vi "Seq Test Editor.vi"(6 "User Name":string="Jon", 8 "Sys Error":errorcluster, 9 "Part Type":string="LX", 10 "Station":string="Audit Station", 11 "Base Path":path=path "C:/Labview Code") -> (0 "Sys Error Out":errorcluster)   [LabVIEW 2018]
uses:
  type defs/Sequence Info.ctl
  type defs/Sequence Status.ctl
  type defs/config paths for seq def.ctl
  <vilib>/Utility/miscctls.llb/LVRowAndColumnUnsignedTypeDef.ctl
  <vilib>/Utility/file.llb/Write To Spreadsheet File (string).vi
panel:
  in  "Save":bool
  out "Sequence Name":string="F15 Audit 1 Sequence"
  in  "Exit":bool
  in  "Sequence":i32(listbox)=7
  in  "Steps":i32(listbox)
  in  "Edit Step":bool
  in  "Up":bool
  in  "Down":bool
  in  "Copy Step":bool
  in  "Delete":bool
  in  "Insert Step":bool
  # "[Page Up]"
  # "[Page Dn]"
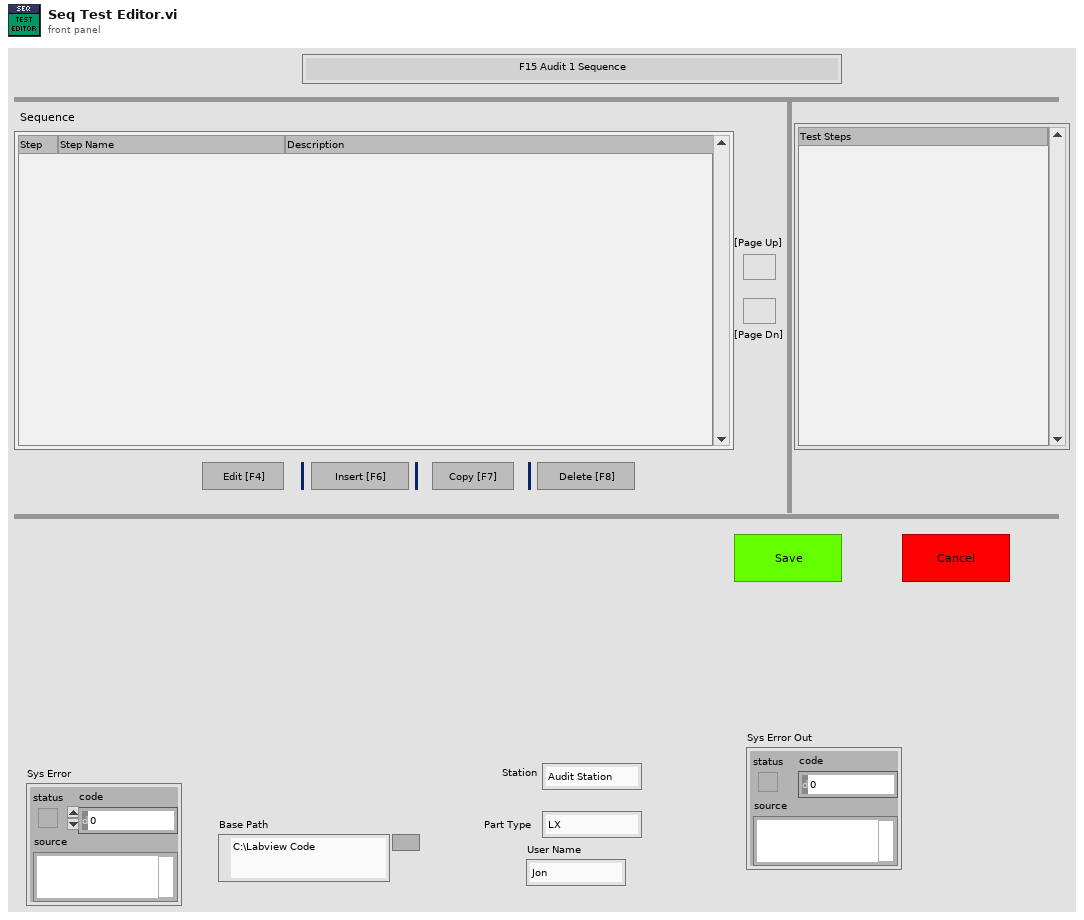
[diagram p1: front panel]
types:
  T1 = typedef "Sequence Status.ctl" = enum16{"No Change", "Edited", "New Step", "Deleted", "Moved Up", "Moved Down", "Copied"}
  T2 = typedef "Sequence Info.ctl" = cluster{"Name":string, "Description":string, "data string":string}
  T3 = cluster{"Type":string, "Sequence Name:":i32, "Sequence":refnum<vi>, "Steps":refnum<vi>, "Sequence Info":T2[], "Sequence Scroll":u32, "Basic Steps":string[], "Sequences":string[], "Sequence Text":string, "appended path":path, "Station":string, "New Step?":bool, "Part Type":string, "User Name":string, "Sequence History":string[][], "Sequence Status":T1, "Sequence History Index":i32, "Step History Data":string[], "VI Names":string[], "Sys Error":errorcluster, "Current Sequence":string[][], "Sequence Path":path, "Base Path":path}
  T4 = enum8{"Enabled", "Disabled", "Disabled and Grayed Out"}
  T5 = typedef "config paths for seq def.ctl" = cluster{"Part Type":string, "base path":path}
  T6 = typedef "LVRowAndColumnUnsignedTypeDef.ctl" = cluster{"Row":u32, "Column":u32}
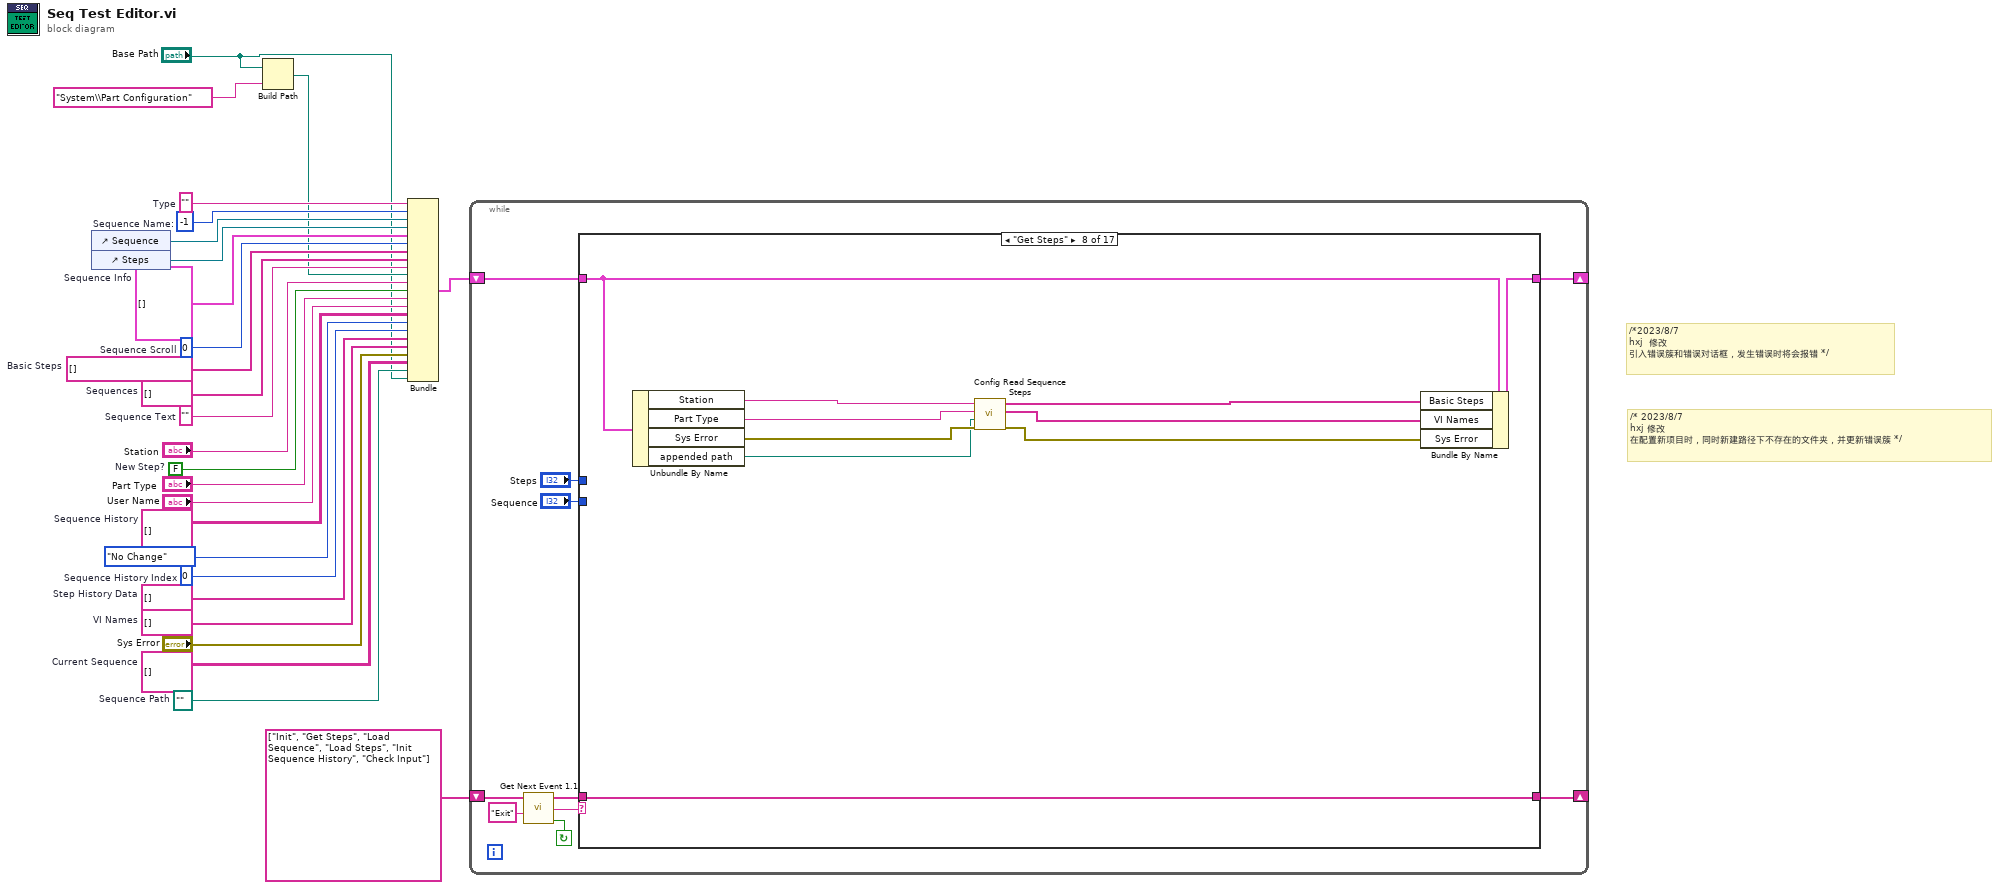
[diagram p0: block diagram]
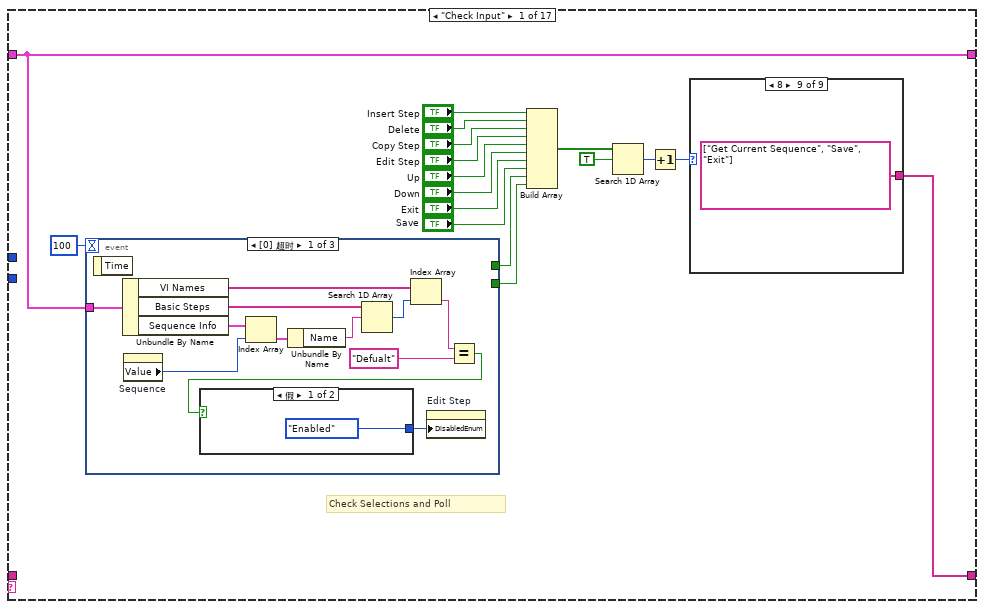
[diagram p2: hidden frame]
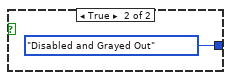
[diagram p3: hidden frame]
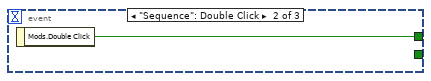
[diagram p4: hidden frame]
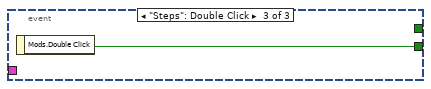
[diagram p5: hidden frame]
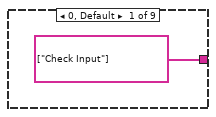
[diagram p6: hidden frame]
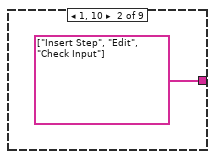
[diagram p7: hidden frame]
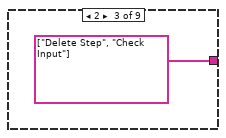
[diagram p8: hidden frame]
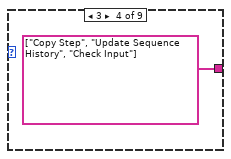
[diagram p9: hidden frame]
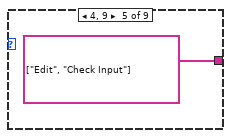
[diagram p10: hidden frame]
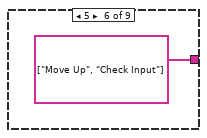
[diagram p11: hidden frame]
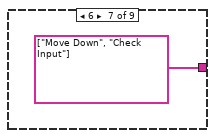
[diagram p12: hidden frame]
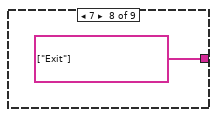
[diagram p13: hidden frame]
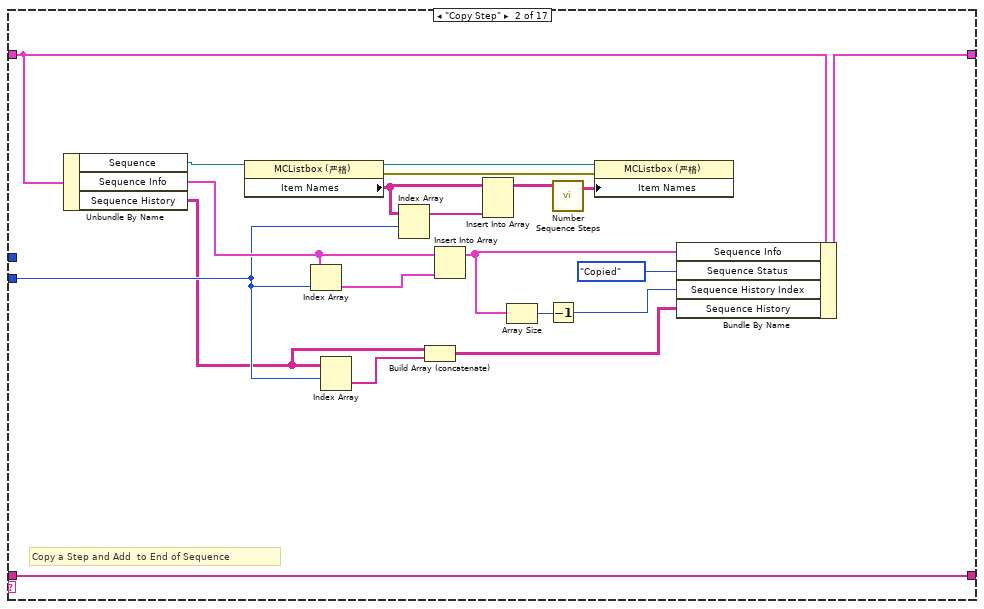
[diagram p14: hidden frame]
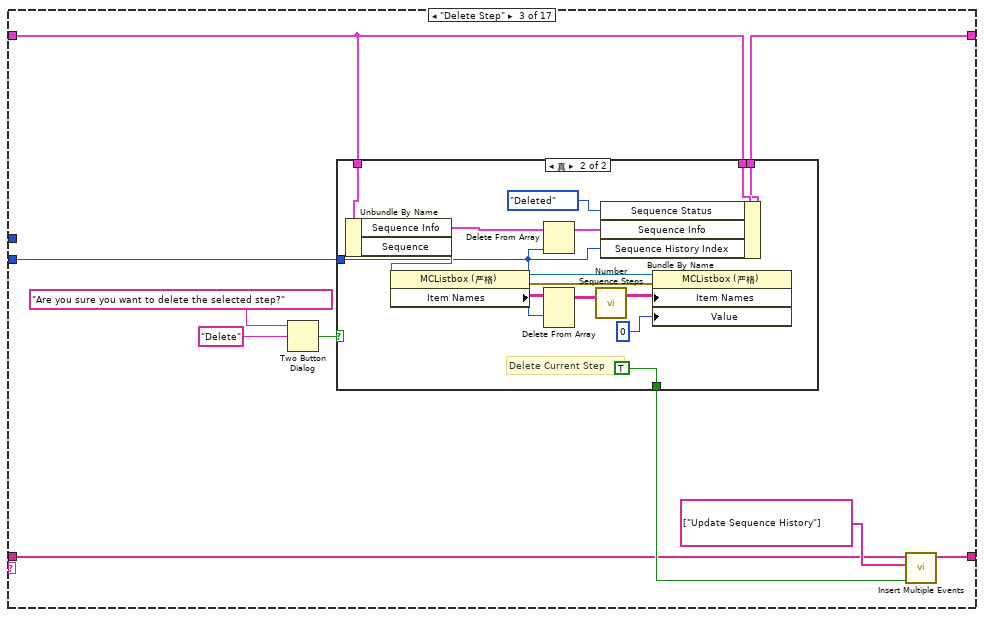
[diagram p15: hidden frame]
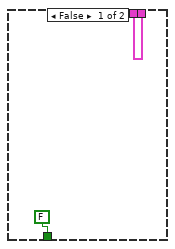
[diagram p16: hidden frame]
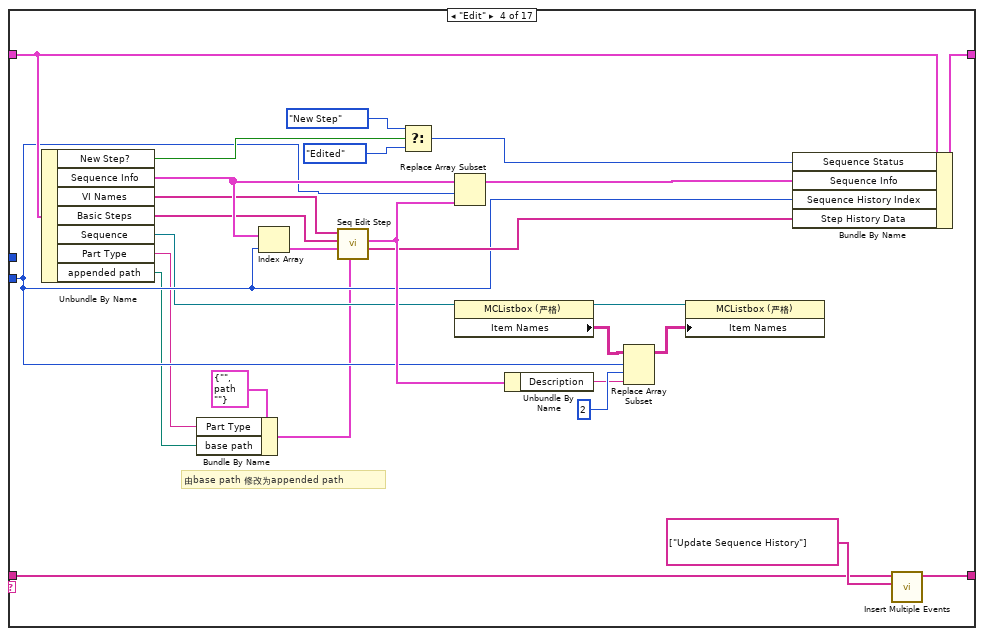
[diagram p17: hidden frame]
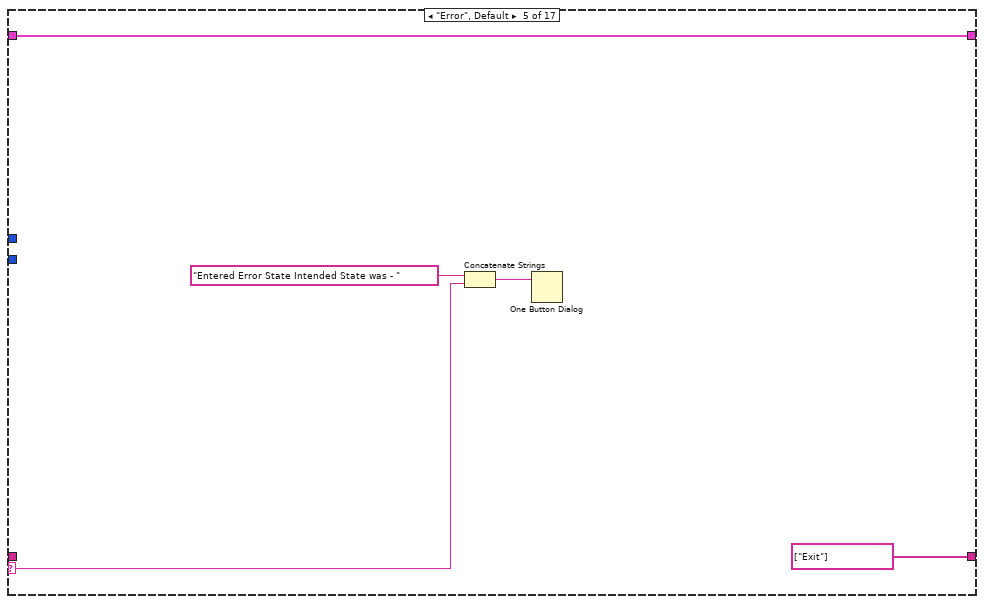
[diagram p18: hidden frame]
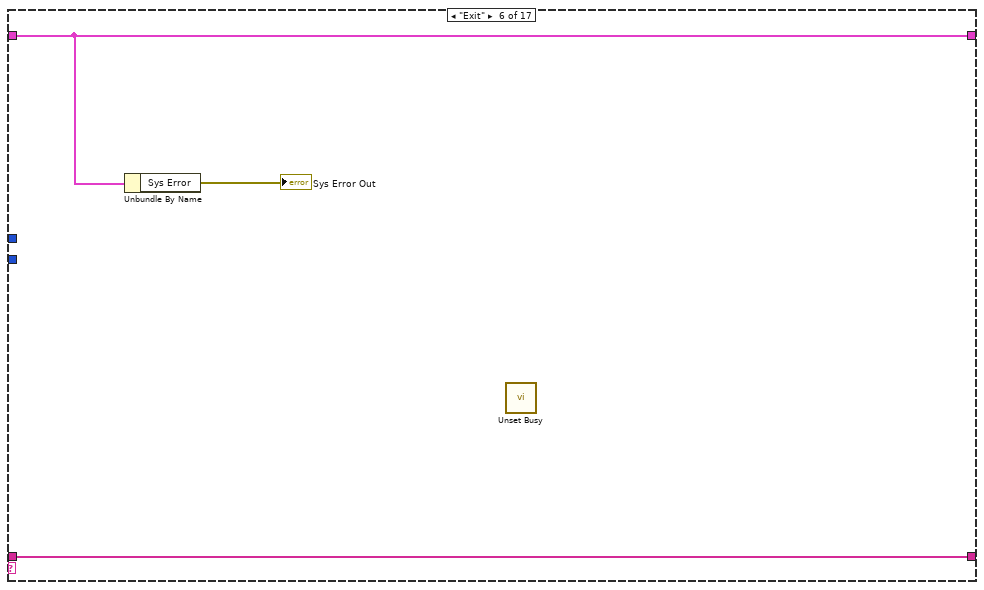
[diagram p19: hidden frame]
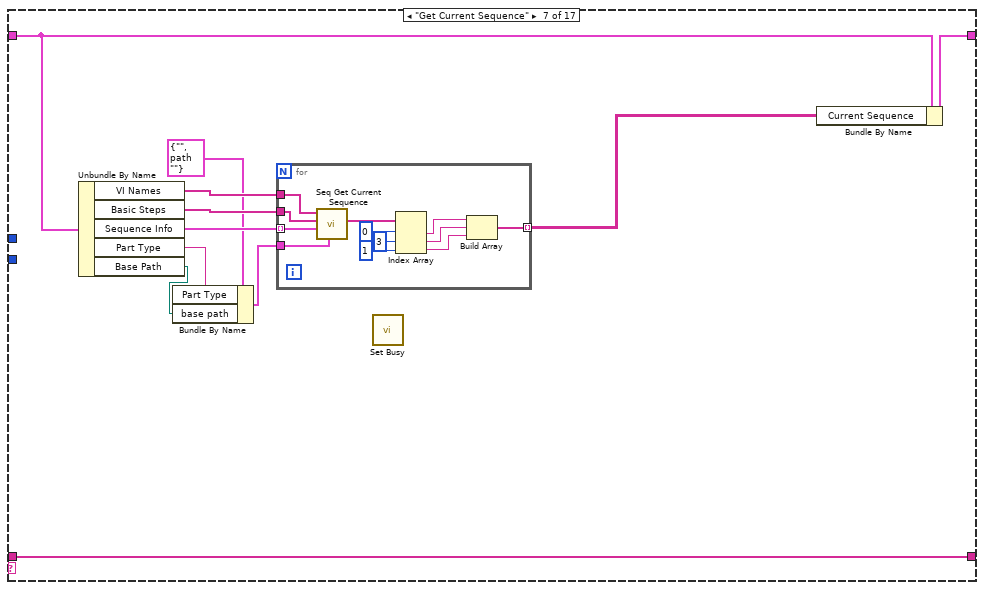
[diagram p20: hidden frame]
diagram:
  w4 = path ""  # Sequence Path
  w5 = string[][] []  # Current Sequence
  w7 = string[] []  # VI Names
  w8 = string[] []  # Step History Data
  w9 = 0  # Sequence History Index
  w16 = FALSE  # New Step?
  w11 = string[][] []  # Sequence History
  w14 = T2[] []  # Sequence Info
  w18 = string[] []  # Sequences
  w20 = ""  # Sequence Text
  w21 = -1  # Sequence Name:
  w17 = string[] []  # Basic Steps
  w23 = u32 0  # Sequence Scroll
  w19 = ""  # Type
  # "/* 2023/8/7\nhxj 修改\n在配置新项目时，同时新建路径下不存在的文件夹，并更新错误簇 */"
  # "/*2023/8/7\nhxj  修改\n引入错误簇和错误对话框，发生错误时将会报错 */"
  n1 = control-ref of="Sequence"() -> (w24:refnum<vi>)
  n2 = control-ref of="Steps"() -> (w22:refnum<vi>)
  n3 = Build Path(base path="Base Path", name or relative path="System\\Part Configuration" ("string")) -> (appended path=w3:path)
  n4 = Bundle("Type"=w19, "Sequence Name:"=w21, "Sequence"=w24, "Steps"=w22, "Sequence Info"=w14, "Sequence Scroll"=w23, "Basic Steps"=w17, "Sequences"=w18, "Sequence Text"=w20, "appended path"=w3, "Station"="Station", "New Step?"=w16, "Part Type"="Part Type", "User Name"="User Name", "Sequence History"=w11, "Sequence Status"=Sequence_Status."No Change", "Sequence History Index"=w9, "Step History Data"=w8, "VI Names"=w7, "Sys Error"="Sys Error", "Current Sequence"=w5, "Sequence Path"=w4, "Base Path"="Base Path") -> (w25:T3)  [unwired: 1 in]
  n5 = while {
    shift-right: [w36] -> _
    shift-left: string[] ["Init", "Get Steps", "Load Sequence", "Load Steps", "Init Sequence History", "Check Input"] -> [w33]
    shift-right: [w34] -> _
    shift-left: w25 -> [w35]
    stop <- w30 continue-if-true
    n6 = call "Get Next Event 1.1.vi"("Exit Event"="Exit", "event queue in"=w33) -> ("Condition (Exit:F)"=w30:bool, "next event"=w31:string, "event queue out"=w32:string[])  [unwired: 6 in, 1 out]
    n7 = case shown="\"Get Steps\"" w31 {
      selector: w31 -> [_ _ _ _ w154 _ _ _ _ _ _ _ _ _ _ _ _]
      tunnel: w32 -> [_ w91 w99 w133 _ w160 w171 w193 w202 w217 w230 w265 w273 w275 w311 w346 w402]
      tunnel: [w46 w91 w100 w134 string[] ["Exit"] ("event queue out") w160 w171 w193 w202 w217 w230 w265 w273 w276 w310 w346 w402] -> w36
      tunnel: w35 -> [w37 w93 w105 w152 w157 w159 w167 w192 w196 w207 w241 w263 w268 w286 w313 w338 w399]
      tunnel: [w37 w92 w104 w151 w157 w159 w166 w191 w196 w206 w240 w267 w268 w288 w315 w337 w401] -> w34
      tunnel: "Steps" -> [_ _ _ _ _ _ _ _ _ _ w234 _ _ _ _ _ _]
      tunnel: "Sequence" -> [_ w83 w103 w136 _ _ _ _ _ _ w229 _ _ w280 w314 _ _]
      frame "Check Input" {
        # "Check Selections and Poll"
        n8 = event shown="[0] 超时" {
          selector: _ -> [_ _ _]
          dyn-events: _ -> [_ _ _]
          timeout: 100 -> [_ _ _]
          tunnel: [_ w68 _] -> w43
          tunnel: [_ _ w69] -> w42
          tunnel: w37 -> [w65 _ _]
          event Timeout {
            n9 = event-data() -> ()  [unwired: 1 in, 1 out]
            n10 = Unbundle By Name(w65) -> ("VI Names"=w60:string[], "Basic Steps"=w62:string[], "Sequence Info"=w64:T2[])
            n11 = property on="Sequence" class="MCListbox (严格)"() -> ("Value"=w54:i32)  [unwired: 2 in, 2 out]
            n12 = Index Array(array=w64, index=w54) -> (element=w63:T2)
            n13 = Unbundle By Name(w63) -> ("Name"=w61:string)
            n14 = Search 1D Array(1D array=w62, element=w61) -> (index of element=w59:i32)  [unwired: 1 in]
            n15 = Index Array(array=w60, index=w59) -> (element=w57:string)
            n16 = Equal?(x=w57, y="Defualt") -> (x = y?=w56:bool)
            n17 = case shown="假" w56 {
              tunnel: [T4."Enabled" ("禁用") T4."Disabled and Grayed Out" ("禁用")] -> w55
              frame False {
              }
              frame True {
              }
            }
            n18 = property on="Edit Step" class="Bool"("DisabledEnum"=w55) -> ()  [unwired: 2 in, 2 out]
          }
          event "Sequence": Double Click {
            n19 = event-data() -> ("Mods.Double Click"=w68:bool)  [unwired: 1 in]
          }
          event "Steps": Double Click {
            n20 = event-data() -> ("Mods.Double Click"=w69:bool)  [unwired: 1 in]
          }
        }
        n21 = Build Array("Insert Step", "Delete", "Copy Step", "Edit Step", "Up", "Down", "Exit", "Save", w43, w42) -> (w49:bool[])
        n22 = Search 1D Array(1D array=w49, element=TRUE) -> (index of element=w48:i32)  [unwired: 1 in]
        n23 = Increment(x=w48) -> (x+1=w38:i32)
        n24 = case shown="8" w38 {
          tunnel: [string[] ["Check Input"] string[] ["Insert Step", "Edit", "Check Input"] string[] ["Delete Step", "Check Input"] string[] ["Copy Step", "Update Sequence History", "Check Input"] string[] ["Edit", "Check Input"] string[] ["Move Up", "Check Input"] string[] ["Move Down", "Check Input"] string[] ["Exit"] string[] ["Get Current Sequence", "Save", "Exit"]] -> w46
          frame 0, Default {
          }
          frame 1, 10 {
          }
          frame 2 {
          }
          frame 3 {
          }
          frame 4, 9 {
          }
          frame 5 {
          }
          frame 6 {
          }
          frame 7 {
          }
          frame 8 {
          }
        }
      }
      frame "Copy Step" {
        # "Copy a Step and Add  to End of Sequence"
        n25 = Unbundle By Name(w93) -> ("Sequence"=w98:refnum<vi>, "Sequence Info"=w88:T2[], "Sequence History"=w82:string[][])
        n26 = property class="MCListbox (严格)"(reference=w98) -> (reference out=w95:refnum<vi>, error out=w94:errorcluster, "Item Names"=w90:string[][])  [unwired: 1 in]
        n27 = Index Array(array=w88, index=w83) -> (element=w87:T2)
        n28 = Index Array(array=w82, index (row)=w83) -> (element=w81:string[])  [unwired: 1 in]
        n29 = Index Array(array=w90, index (row)=w83) -> (element=w89:string[])  [unwired: 1 in]
        n30 = Build Array (concatenate)(w82, w81) -> (w80:string[][])
        n31 = Insert Into Array(array=w88, new element=w87) -> (w79:T2[])  [unwired: 1 in]
        n32 = Insert Into Array(array=w90, new element=w89) -> (w97:string[][])  [unwired: 2 in]
        n33 = Array Size(array=w79) -> (size(s)=w85:i32)
        n34 = Decrement(x=w85) -> (x-1=w84:i32)
        n35 = call "Number Sequence Steps.vi"("Sequence Names"=w97) -> ("ItemNames Out"=w96:string[][])  [unwired: 1 out]
        n36 = property class="MCListbox (严格)"(reference=w95, error in=w94, "Item Names"=w96) -> ()  [unwired: 2 out]
        n37 = Bundle By Name(cluster=w93, "Sequence Info"=w79, "Sequence Status"=Sequence_Status."Copied", "Sequence History Index"=w84, "Sequence History"=w80) -> (w92:T3)
      }
      frame "Delete Step" {
        n38 = Two Button Dialog(message="Are you sure you want to delete the selected step?", 2:"Delete" ("T button name (\"OK\")")) -> (T button?=w106:bool)  [unwired: 1 in]
        n39 = case shown="真" w106 {
          tunnel: w105 -> [_ w125]
          tunnel: w105 -> [w110 w123]
          tunnel: [w110 w122] -> w104
          tunnel: w103 -> [_ w112]
          tunnel: [FALSE TRUE] -> w101
          frame False {
          }
          frame True {
            # "Delete Current Step"
            n40 = Unbundle By Name(w125) -> ("Sequence Info"=w121:T2[], "Sequence"=w124:refnum<vi>)
            n41 = property class="MCListbox (严格)"(reference=w124) -> (reference out=w118:refnum<vi>, error out=w117:errorcluster, "Item Names"=w119:string[][])  [unwired: 1 in]
            n42 = Delete From Array(array=w121, index=w112) -> (array with subset deleted=w120:T2[])  [unwired: 1 in, 1 out]
            n43 = Delete From Array(array=w119, index (row)=w112) -> (array with subset deleted=w116:string[][])  [unwired: 2 in, 1 out]
            n44 = call "Number Sequence Steps.vi"("Sequence Names"=w116) -> ("ItemNames Out"=w115:string[][])  [unwired: 1 out]
            n45 = Bundle By Name(cluster=w123, "Sequence Status"=Sequence_Status."Deleted", "Sequence Info"=w120, "Sequence History Index"=w112) -> (w122:T3)
            n46 = property class="MCListbox (严格)"(reference=w118, error in=w117, "Item Names"=w115, "Value"=0) -> ()  [unwired: 2 out]
          }
        }
        n47 = call "Insert Multiple Events.vi"("Insert all? (T)"=w101, "Events to Insert"=string[] ["Update Sequence History"], "Event queue in"=w99) -> ("Event queue out"=w100:string[])  [unwired: 4 in]
      }
      frame "Edit" {
        # "由base path 修改为appended path"
        n48 = Unbundle By Name(w152) -> ("New Step?"=w141:bool, "Sequence Info"=w149:T2[], "VI Names"=w132:string[], "Basic Steps"=w130:string[], "Sequence"=w131:refnum<vi>, "Part Type"=w128:string, "appended path"=w126:path)
        n49 = Bundle By Name(cluster=T5 {"Part Type"="", "base path"=path ""} ("config paths"), "Part Type"=w128, "base path"=w126) -> (w127:T5)
        n50 = Index Array(array=w149, index=w136) -> (element=w142:T2)
        n51 = call "Seq Edit Step.vi"("config paths"=w127, "Segment Info In"=w142, "Basic Steps"=w130, "VI Names"=w132) -> ("Step Hisitory"=w137:string[], "Segment Info Out"=w148:T2)  [unwired: 4 in, 2 out]
        n52 = Select(t=Sequence_Status."New Step" ("Sequence Status"), s=w141, f=Sequence_Status."Edited" ("Sequence Status")) -> (s? t:f=w138:T1)
        n53 = Replace Array Subset(array=w149, new element=w148, index=w136) -> (w150:T2[])
        n54 = property class="MCListbox (严格)"(reference=w131) -> (reference out=w146:refnum<vi>, "Item Names"=w147:string[][])  [unwired: 1 in, 1 out]
        n55 = Unbundle By Name(w148) -> ("Description"=w144:string)
        n56 = Replace Array Subset(array=w147, new element=w144, index (row)=w136, index (col)=2 ("disabled index (col)")) -> (w143:string[][])
        n57 = property class="MCListbox (严格)"(reference=w146, "Item Names"=w143) -> ()  [unwired: 1 in, 2 out]
        n58 = Bundle By Name(cluster=w152, "Sequence Status"=w138, "Sequence Info"=w150, "Sequence History Index"=w136, "Step History Data"=w137) -> (w151:T3)
        n59 = call "Insert Multiple Events.vi"("Events to Insert"=string[] ["Update Sequence History"], "Event queue in"=w133) -> ("Event queue out"=w134:string[])  [unwired: 5 in]
      }
      frame "Error", Default {
        n60 = Concatenate Strings("Entered Error State Intended State was - " ("string"), w154) -> (w153:string)
        n61 = One Button Dialog(message=w153) -> ()  [unwired: 1 in, 1 out]
      }
      frame "Exit" {
        n62 = Unbundle By Name(w159) -> ("Sys Error"=→"Sys Error Out":errorcluster)
        n63 = call <vilib>:"Unset Busy.vi"() -> ()  [unwired: 11 in, 1 out]
      }
      frame "Get Current Sequence" {
        n64 = Unbundle By Name(w167) -> ("VI Names"=w168:string[], "Basic Steps"=w169:string[], "Sequence Info"=w170:T2[], "Part Type"=w163:string, "Base Path"=w162:path)
        n65 = Bundle By Name(cluster=T5 {"Part Type"="", "base path"=path ""} ("config paths"), "Part Type"=w163, "base path"=w162) -> (w161:T5)
        n66 = for {
          tunnel: w170 -> [w183] mode=indexing
          tunnel: w169 -> [w182]
          tunnel: w168 -> [w181]
          tunnel: [w176] -> w165 mode=indexing
          tunnel: w161 -> [w172]
          n67 = call "Seq Get Current Sequence.vi"("config paths"=w172, "Segment Info In"=w183, "Basic Steps"=w182, "VI Names"=w181) -> ("Step Hisitory"=w180:string[])  [unwired: 6 in, 1 out]
          n68 = Index Array(array=w180, index #1=0 ("index"), index #2=3 ("index"), index #3=1 ("index")) -> (element #1=w179:string, element #2=w178:string, element #3=w177:string)
          n69 = Build Array(w179, w178, w177) -> (w176:string[])
        }
        n70 = call <vilib>:"Set Busy.vi"() -> ()  [unwired: 10 in, 2 out]
        n71 = Bundle By Name(cluster=w167, "Current Sequence"=w165) -> (w166:T3)
      }
      frame "Get Steps" {
        n72 = Unbundle By Name(w192) -> ("Station"=w189:string, "Part Type"=w190:string, "Sys Error"=w186:errorcluster, "appended path"=w184:path)
        n73 = call "Config Read Sequence Steps.vi"("Error In"=w186, "Base Path"=w184, "Part Type"=w190, "Station Name"=w189) -> ("Error Out"=w185:errorcluster, "VI Names"=w187:string[], "Sequence Steps"=w188:string[])  [unwired: 5 in]
        n74 = Bundle By Name(cluster=w192, "Basic Steps"=w188, "VI Names"=w187, "Sys Error"=w185) -> (w191:T3)
      }
      frame "Init" {
        w199 = string[][] [] ("Item Names")
        w198 = u32 0
        w195 = 0 ("Value")
        n75 = Unbundle By Name(w196) -> ("Sequence"=w201:refnum<vi>, "Steps"=w200:refnum<vi>)
        n76 = property class="MCListbox (严格)"(reference=w201, "Item Names"=w199, "Value"=w195, "Selection Color"=w198) -> ()  [unwired: 1 in, 2 out]
        n77 = property class="MCListbox (严格)"(reference=w200, "Item Names"=w199, "Value"=w195, "Selection Color"=w198, "Disabled Items"=i32[] [], "TopLeft"=T6 {"Row"=0, "Column"=0} ("左上可见单元格")) -> ()  [unwired: 1 in, 2 out]
      }
      frame "Init Sequence History" {
        n78 = Unbundle By Name(w207) -> ("User Name"=w211:string, "Part Type"=w213:string, "Station"=w215:string, "Sequence Info"=w216:T2[], "Sequence Status"=w204:T1)
        n79 = Get Date/Time String() -> (date string=w209:string, time string=w210:string)  [unwired: 3 in]
        n80 = Format Into String(w213) -> (resulting string=w212:string)  [unwired: 3 in, 1 out]
        n81 = Format Into String(w215) -> (resulting string=w214:string)  [unwired: 3 in, 1 out]
        n82 = Format Into String(w204) -> (resulting string=w208:string)  [unwired: 3 in, 1 out]
        n83 = for {
          tunnel: w216 -> [w227] mode=indexing
          tunnel: w214 -> [w222]
          tunnel: w212 -> [w223]
          tunnel: w211 -> [w224]
          tunnel: w210 -> [w225]
          tunnel: w209 -> [w226]
          tunnel: [w220] -> w205 mode=indexing
          tunnel: w208 -> [w219]
          tunnel: "NA" -> [w218]
          n84 = Unbundle By Name(w227) -> ("Name"=w221:string)
          n85 = Build Array(w224, w226, w225, w223, w222, w221, w219, w218, w218) -> (w220:string[])
        }
        n86 = Bundle By Name(cluster=w207, "Sequence History"=w205) -> (w206:T3)
      }
      frame "Insert Step" {
        n87 = Unbundle By Name(w241) -> ("Sequence"=w249:refnum<vi>, "Steps"=w252:refnum<vi>, "Sequence Info"=w236:T2[])
        n88 = property class="MCListbox (严格)"(reference=w252) -> (error out=w248:errorcluster, "Item Names"=w251:string[][])  [unwired: 1 in, 1 out]
        n89 = case shown="..-1" w229 {
          selector: w229 -> [w253 _]
          tunnel: [w253 0 ("Sequence")] -> w228
          frame 0.. {
          }
          frame ..-1 {
          }
        }
        n90 = Index Array(array=w251, index (row)=w234, index (col)=0 ("disabled index (col)")) -> (element=w235:string)
        n91 = property class="MCListbox (严格)"(reference=w249, error in=w248) -> (reference out=w243:refnum<vi>, error out=w242:errorcluster, "Item Names"=w246:string[][])
        n92 = Bundle By Name(cluster=T2 {"Name"="", "Description"="", "data string"=""} ("Segment Data"), "Name"=w235) -> (w238:T2)
        n93 = Build Array("1" ("element"), w235, "") -> (w245:string[])
        n94 = Insert Into Array(array=w246, index (row)=w228, new element=w245) -> (w247:string[][])  [unwired: 1 in]
        n95 = Insert Into Array(array=w236, index=w228, new element=w238) -> (w237:T2[])
        n96 = call "Number Sequence Steps.vi"("Sequence Names"=w247) -> ("ItemNames Out"=w244:string[][])  [unwired: 1 out]
        n97 = property class="MCListbox (严格)"(reference=w243, error in=w242, "Item Names"=w244, "Value"=w228) -> ()  [unwired: 2 out]
        n98 = Bundle By Name(cluster=w241, "Sequence Info"=w237, "New Step?"=TRUE) -> (w240:T3)
      }
      frame "Load Sequence" {
        # "Load Sequence"
        n99 = Unbundle By Name(w263) -> ("Sequence"=w266:refnum<vi>, "Part Type"=w259:string, "Station"=w260:string, "appended path"=w257:path, "Sys Error"=w256:errorcluster)
        n100 = call "Config Load Sequence.vi"("Sys Error In"=w256, "Base Path"=w257, "Station"=w260, "Part Type"=w259) -> ("Sys Error Out"=w255:errorcluster, "Sequence Name"=→"Sequence Name":string, "Item Names"=w264:string[][], "Seqence Info"=w262:T2[], "Sequence Path"=w258:path)  [unwired: 3 in]
        n101 = property class="MCListbox (严格)"(reference=w266, "Item Names"=w264) -> ()  [unwired: 1 in, 2 out]
        n102 = Bundle By Name(cluster=w263, "Sequence Path"=w258, "Sequence Info"=w262, "Sys Error"=w255) -> (w267:T3)
      }
      frame "Load Steps" {
        n103 = Unbundle By Name(w268) -> ("Steps"=w272:refnum<vi>, "Basic Steps"=w271:string[])
        n104 = Build Array(w271) -> (w270:string[][])
        n105 = Transpose 2D Array(2D array=w270) -> (transposed array=w269:string[][])
        n106 = property class="MCListbox (严格)"(reference=w272, "Item Names"=w269) -> ()  [unwired: 1 in, 2 out]
      }
      frame "Move Down" {
        # "Move the step Down one in the sequence"
        n107 = Unbundle By Name(w286) -> ("Sequence Info"=w285:T2[], "Sequence"=w284:refnum<vi>)
        n108 = property class="MCListbox (严格)"(reference=w284) -> (reference out=w289:refnum<vi>, error out=w287:errorcluster, "Item Names"=w283:string[][])  [unwired: 1 in]
        n109 = Array Size(array=w283) -> (size(s)=w282:i32[])
        n110 = Index Array(array=w282) -> (element=w281:i32)  [unwired: 1 in]
        n111 = Decrement(x=w281) -> (x-1=w278:i32)
        n112 = Greater?(x=w278, y=w280) -> (0:w279:bool)
        n113 = case shown="假" w279 {
          tunnel: w289 -> [_ w308]
          tunnel: [w291 w307] -> w288
          tunnel: w287 -> [_ w306]
          tunnel: w286 -> [w291 w305]
          tunnel: w285 -> [_ w304]
          tunnel: w283 -> [_ w300]
          tunnel: w280 -> [_ w293]
          tunnel: [FALSE TRUE] -> w274
          frame False {
            # "At Bottom"
          }
          frame True {
            # "Move Down"
            n114 = Delete From Array(array=w304, index=w293) -> (deleted portion=w302:T2, array with subset deleted=w303:T2[])  [unwired: 1 in]
            n115 = Delete From Array(array=w300, index (row)=w293) -> (deleted portion=w298:string[], array with subset deleted=w299:string[][])  [unwired: 2 in]
            n116 = Increment(x=w293) -> (x+1=w297:i32)
            n117 = Insert Into Array(array=w303, index=w297, new element=w302) -> (w301:T2[])
            n118 = Insert Into Array(array=w299, index (row)=w297, new element=w298) -> (w296:string[][])  [unwired: 1 in]
            n119 = Bundle By Name(cluster=w305, "Sequence Status"=Sequence_Status."Moved Down", "Sequence Info"=w301, "Sequence History Index"=w293) -> (w307:T3)
            n120 = call "Number Sequence Steps.vi"("Sequence Names"=w296) -> ("ItemNames Out"=w295:string[][])  [unwired: 1 out]
            n121 = property class="MCListbox (严格)"(reference=w308, error in=w306, "Item Names"=w295, "Value"=w297) -> ()  [unwired: 2 out]
          }
        }
        n122 = call "Insert Multiple Events.vi"("Insert all? (T)"=w274, "Events to Insert"=string[] ["Update Sequence History"], "Event queue in"=w275) -> ("Event queue out"=w276:string[])  [unwired: 4 in]
      }
      frame "Move Up" {
        # "Move the Step Up one in the Sequence"
        n123 = case shown="1, 默认" w314 {
          selector: w314 -> [_ w319]
          tunnel: [w317 w335] -> w315
          tunnel: w313 -> [w317 w325]
          tunnel: w313 -> [_ w324]
          tunnel: [FALSE TRUE] -> w309
          frame 0 {
            # "Do Not Move Up If at Top"
          }
          frame 1, Default {
            # "Move Up"
            n124 = Unbundle By Name(w324) -> ("Sequence Info"=w333:T2[], "Sequence"=w331:refnum<vi>)
            n125 = property class="MCListbox (严格)"(reference=w331) -> (reference out=w336:refnum<vi>, error out=w334:errorcluster, "Item Names"=w328:string[][])  [unwired: 1 in]
            n126 = Delete From Array(array=w333, index=w319) -> (deleted portion=w330:T2, array with subset deleted=w332:T2[])  [unwired: 1 in]
            n127 = Delete From Array(array=w328, index (row)=w319) -> (deleted portion=w326:string[], array with subset deleted=w327:string[][])  [unwired: 2 in]
            n128 = Decrement(x=w319) -> (x-1=w320:i32)
            n129 = Insert Into Array(array=w332, index=w320, new element=w330) -> (w329:T2[])
            n130 = Insert Into Array(array=w327, index (row)=w320, new element=w326) -> (w323:string[][])  [unwired: 1 in]
            n131 = Bundle By Name(cluster=w325, "Sequence Status"=Sequence_Status."Moved Up", "Sequence Info"=w329, "Sequence History Index"=w319) -> (w335:T3)
            n132 = call "Number Sequence Steps.vi"("Sequence Names"=w323) -> ("ItemNames Out"=w322:string[][])  [unwired: 1 out]
            n133 = property class="MCListbox (严格)"(reference=w336, error in=w334, "Item Names"=w322, "Value"=w320) -> ()  [unwired: 2 out]
          }
        }
        n134 = call "Insert Multiple Events.vi"("Insert all? (T)"=w309, "Events to Insert"=string[] ["Update Sequence History"], "Event queue in"=w311) -> ("Event queue out"=w310:string[])  [unwired: 4 in]
      }
      frame "Save" {
        n135 = Unbundle By Name(w338) -> ("Sequence Path"=w344:path, "Sequence Info"=w343:T2[], "Sequence History"=w342:string[][], "Part Type"=w341:string, "Station"=w340:string, "Current Sequence"=w345:string[][], "appended path"=w339:path)
        n136 = disable-structure shown="启用" {
          disable-tunnel: w345 -> [w364 w378]
          disable-tunnel: w344 -> [w363 w392]
          disable-tunnel: w343 -> [w362 w384]
          disable-tunnel: w342 -> [w360 w387]
          disable-tunnel: w341 -> [w354 w391]
          disable-tunnel: w340 -> [w353 w390]
          disable-tunnel: w339 -> [_ w377]
          disable-tunnel: w338 -> [w347 w376]
          disable-tunnel: [w347 w374] -> w337
          frame Disabled {
            w361 = path "C:/Labview Code" ("Base Path 2")
            n137 = Flatten To String(anything=w362) -> (data string=w373:string)  [unwired: 3 in, 2 out]
            n138 = call "Write Characters To File with Advisory Dialog Option.vi"("character string"=w373, "file path (dialog if empty)"=w363) -> ()  [unwired: 8 in, 2 out]
            n139 = call <vilib>:"Space Constant.vi"() -> ("String"=w352:string)
            n140 = call <vilib>:"Space Constant.vi"() -> ("String"=w351:string)
            n141 = Concatenate Strings("System\\Part Configuration\\" ("name or relative path"), w354, "\\Sequences History\\" ("name or relative path"), w353, "\\" ("name or relative path"), w354, w352, w353, " Sequences History.txt" ("string")) -> (w371:string)
            n142 = Concatenate Strings("System\\Part Configuration\\" ("name or relative path"), w354, "\\Current Sequences\\" ("name or relative path"), w353, "\\" ("name or relative path"), w354, w351, w353, " Current Sequences.txt" ("string")) -> (w355:string)
            n143 = Build Array("\n") -> (w367:string[])
            n144 = Build Array (concatenate)(w360, w367) -> (w365:string[][])
            n145 = Build Path(base path=w361, name or relative path=w371) -> (appended path=w370:path)
            n146 = Build Path(base path=w361, name or relative path=w355) -> (appended path=w366:path)
            n147 = call-poly <vilib>:"Write To Spreadsheet File.vi"("append to file? (new file:F)"=TRUE, "2D data"=w365, "file path (dialog if empty)"=w370) -> ()  [unwired: 5 in, 1 out]
            n148 = call-poly <vilib>:"Write To Spreadsheet File.vi"("2D data"=w364, "file path (dialog if empty)"=w366) -> ()  [unwired: 6 in, 1 out]
          }
          frame Enabled {
            n149 = Build Array("\n") -> (w389:string[])
            n150 = Build Array (concatenate)(w387, w389) -> (w379:string[][])
            n151 = call "path check.vi"("Base Path"=w377, "Station"=w390, "Patr Type"=w391, "Sequence Path"=w392) -> ("out path"=w385:path[])  [unwired: 6 in, 1 out]
            n152 = Index Array(array=w385) -> (element #1=w383:path, element #2=w381:path, element #3=w380:path)  [unwired: 3 in]
            n153 = Flatten To String(anything=w384) -> (data string=w386:string)  [unwired: 3 in, 2 out]
            n154 = call-poly <vilib>:"Write To Spreadsheet File.vi"("append to file? (new file:F)"=TRUE, "2D data"=w379, "file path (dialog if empty)"=w381) -> ()  [unwired: 5 in, 1 out]
            n155 = call-poly <vilib>:"Write To Spreadsheet File.vi"("2D data"=w378, "file path (dialog if empty)"=w380) -> ()  [unwired: 6 in, 1 out]
            n156 = call "Write Characters To File with Advisory Dialog Option.vi"("character string"=w386, "file path (dialog if empty)"=w383) -> ("error out"=w375:errorcluster)  [unwired: 8 in, 1 out]
            n157 = Bundle By Name(cluster=w376, "Sys Error"=w375) -> (w374:T3)
          }
        }
      }
      frame "Update Sequence History" {
        n158 = Unbundle By Name(w399) -> ("Sequence History"=w398:string[][], "Sequence Status"=w394:T1, "Sequence History Index"=w397:i32, "Step History Data"=w396:string[])
        n159 = Format Into String(w394) -> (resulting string=w393:string)  [unwired: 3 in, 1 out]
        n160 = case shown="\"Edited\"" w394 {
          tunnel: w398 -> [w403 w407 w425 w441 w450 w460 w468]
          tunnel: w397 -> [_ w406 w424 w440 w449 w459 w467]
          tunnel: w396 -> [_ w415 w432 _ _ _ _]
          tunnel: [w403 w405 w423 w439 w448 w453 w461] -> w395
          tunnel: w393 -> [_ w404 w418 w437 w446 w456 w464]
          frame "No Change", Default {
          }
          frame "Edited" {
            n161 = Index Array(array=w407, index (row)=w406) -> (element=w417:string[])  [unwired: 1 in]
            n162 = Index Array(array=w415) -> (element #2=w410:string, element #3=w409:string)  [unwired: 3 in, 1 out]
            n163 = Replace Array Subset(array=w417, new element=w404, index=6) -> (w414:string[])
            n164 = Replace Array Subset(array=w414, new element=w410, index=7) -> (w413:string[])
            n165 = Replace Array Subset(array=w413, new element=w409, index=8) -> (w408:string[])
            n166 = Replace Array Subset(array=w407, new element=w408, index (row)=w406) -> (w405:string[][])  [unwired: 1 in]
          }
          frame "New Step" {
            n167 = Index Array(array=w425, index (row)=w424) -> (element=w434:string[])  [unwired: 1 in]
            n168 = Index Array(array=w432) -> (element #1=w419:string, element #2=w428:string, element #3=w427:string)  [unwired: 3 in]
            n169 = Replace Array Subset(array=w434, new element=w418, index=6) -> (w421:string[])
            n170 = Replace Array Subset(array=w421, new element=w419, index=5) -> (w420:string[])
            n171 = Replace Array Subset(array=w420, new element=w428, index=7) -> (w431:string[])
            n172 = Replace Array Subset(array=w431, new element=w427, index=8) -> (w426:string[])
            n173 = Insert Into Array(array=w425, index (row)=w424, new element=w426) -> (w423:string[][])  [unwired: 1 in]
          }
          frame "Moved Up" {
            n174 = Delete From Array(array=w441, index (row)=w440) -> (deleted portion=w438:string[], array with subset deleted=w443:string[][])  [unwired: 2 in]
            n175 = Replace Array Subset(array=w438, new element=w437, index=6) -> (w435:string[])
            n176 = Decrement(x=w440) -> (x-1=w442:i32)
            n177 = Insert Into Array(array=w443, index (row)=w442, new element=w435) -> (w439:string[][])  [unwired: 1 in]
          }
          frame "Moved Down" {
            n178 = Delete From Array(array=w450, index (row)=w449) -> (deleted portion=w447:string[], array with subset deleted=w452:string[][])  [unwired: 2 in]
            n179 = Replace Array Subset(array=w447, new element=w446, index=6) -> (w444:string[])
            n180 = Increment(x=w449) -> (x+1=w451:i32)
            n181 = Insert Into Array(array=w452, index (row)=w451, new element=w444) -> (w448:string[][])  [unwired: 1 in]
          }
          frame "Deleted" {
            n182 = Delete From Array(array=w460, index (row)=w459) -> (deleted portion=w457:string[], array with subset deleted=w455:string[][])  [unwired: 2 in]
            n183 = Replace Array Subset(array=w457, new element=w456, index=6) -> (w454:string[])
            n184 = Build Array (concatenate)(w455, w454) -> (w453:string[][])
          }
          frame "Copied" {
            n185 = Delete From Array(array=w468, index (row)=w467) -> (deleted portion=w465:string[], array with subset deleted=w463:string[][])  [unwired: 2 in]
            n186 = Replace Array Subset(array=w465, new element=w464, index=6) -> (w462:string[])
            n187 = Build Array (concatenate)(w463, w462) -> (w461:string[][])
          }
        }
        n188 = Bundle By Name(cluster=w399, "New Step?"=FALSE, "Sequence History"=w395) -> (w401:T3)
      }
    }
  }
